vi "Configure Trigger.vi"(4 "Sensitivity (0:High)":i32(ring) items=["High", "Medium", "Low"], 6 "Trigger Slope (0:Positive)":i32(ring) items=["Positive", "Negative"], 7 "Channel (1:Channel 1)":i32(ring)=1 items=["Channel 1"=1, "Channel 2"=2], 8 "error in (no error)":errorcluster, 9 "Trigger Level (50%)":dbl=50.0 format="%#_4g", 10 "Trigger Level Type (0:Percent)":i32(ring) items=["Percent", "Volts"], 11 "VISA resource name":refnum<visa-resource-name>) -> (0 "error out":errorcluster, 3 "VISA resource name out":refnum<visa-resource-name>)   [LabVIEW 2013, in "Counter.lvlib" / "PICOTEST U62XXA series.lvlib"]
doc: "Configures the Trigger Level. If needed, this VI should be called after Configure Measurement. Volt Peak Measurements <B>does not</B> have Trigger functionality."
uses:
  PICOTEST U62XXA series.lvlib
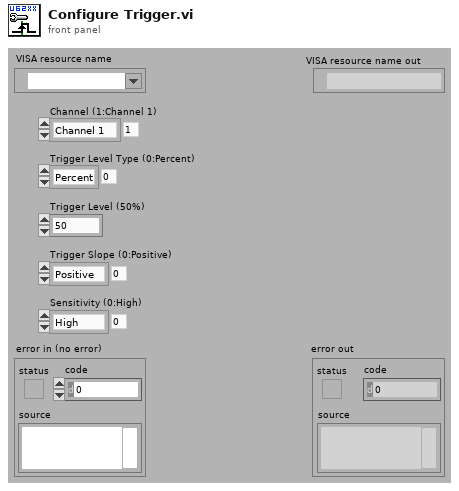
[diagram p1: front panel]
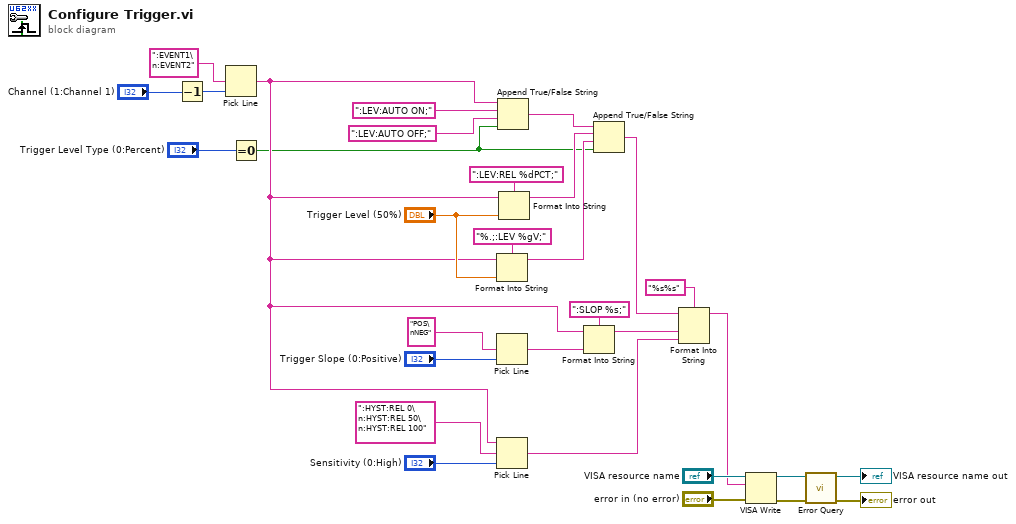
[diagram p0: block diagram]
diagram:
  n1 = Decrement(x="Channel (1:Channel 1)") -> (x-1=w7:i32)
  n2 = Pick Line(multi-line string=":EVENT1\n:EVENT2", line index=w7) -> (output string=w10:string)  [unwired: 1 in]
  n3 = Equal To 0?(x="Trigger Level Type (0:Percent)") -> (x = 0?=w8:bool)
  n4 = Format Into String(format string="%.;:LEV %gV;", initial string=w10, "Trigger Level (50%)") -> (resulting string=w23:string)  [unwired: 1 in, 1 out]
  n5 = Pick Line(multi-line string="POS\nNEG", line index="Trigger Slope (0:Positive)") -> (output string=w14:string)  [unwired: 1 in]
  n6 = Pick Line(string ("")=w10, multi-line string=":HYST:REL 0\n:HYST:REL 50\n:HYST:REL 100", line index="Sensitivity (0:High)") -> (output string=w3:string)
  n7 = Append True/False String(1:w8, 2:":LEV:AUTO OFF;" ("false string"), 3:":LEV:AUTO ON;" ("true string"), 4:w10) -> (0:w26:string)
  n8 = Format Into String(format string=":LEV:REL %dPCT;", initial string=w10, "Trigger Level (50%)") -> (resulting string=w27:string)  [unwired: 1 in, 1 out]
  n9 = Format Into String(format string=":SLOP %s;", initial string=w10, w14) -> (resulting string=w4:string)  [unwired: 1 in, 1 out]
  n10 = Append True/False String(1:w8, 2:w23, 3:w27, 4:w26) -> (0:w5:string)
  n11 = Format Into String(format string="%s%s", initial string=w5, w4, w3) -> (resulting string=w1:string)  [unwired: 1 in, 1 out]
  n12 = VISA Write(VISA resource name="VISA resource name", write buffer=w1, error in (no error)="error in (no error)") -> (VISA resource name out=w20:refnum<visa-resource-name>, error out=w18:errorcluster)  [unwired: 1 out]
  n13 = call "Error Query.vi"("error in (no error)"=w18, "VISA resource name"=w20) -> ("error out"=→"error out":errorcluster, "VISA resource name out"=→"VISA resource name out":refnum<visa-resource-name>)  [unwired: 6 in, 2 out]
